vi "_Serial Write Bit.vi"(1 "BitState(T)":bool=TRUE, 2 "Port type":u8) -> ()   [LabVIEW 2015]
uses:
  <vilib>/rvi/eio/common/nirviEmuTemplateMethod_errors.vi
  <vilib>/eio/EIONode/EIONode.xnode
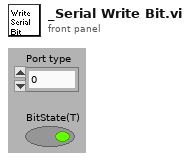
[diagram p1: front panel]
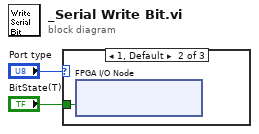
[diagram p0: block diagram]
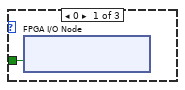
[diagram p2: hidden frame]
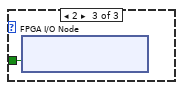
[diagram p3: hidden frame]
diagram:
  n1 = case shown="1, Default" "Port type" {
    tunnel: "BitState(T)" -> [w3 w4 w5]
    frame 0 {
      n2 = xnode "FPGA I/O Node"("Digtal IO/DIO47"=w3) -> ()  [unwired: 1 in, 1 out]
    }
    frame 1, Default {
      n3 = xnode "FPGA I/O Node"("Digtal IO/DIO45"=w4) -> ()  [unwired: 1 in, 1 out]
    }
    frame 2 {
      n4 = xnode "FPGA I/O Node"("Digtal IO/DIO55"=w5) -> ()  [unwired: 1 in, 1 out]
    }
  }
